vi "rozniczka.vi"(5 "dT":dbl format="%#_13g", 7 "u¿yj x0 (T)":bool=TRUE, 9 "Akcja (GET)":T1, 10 "x0":dbl format="%#_13g", 11 "Array in":dbl[](array[numeric])) -> (2 "ostatni":dbl, 3 "Array out":dbl[](array[numeric]))   [LabVIEW 2014]
uses:
  Kontrolki/FVGs/FVG akcje podstawowa.ctl
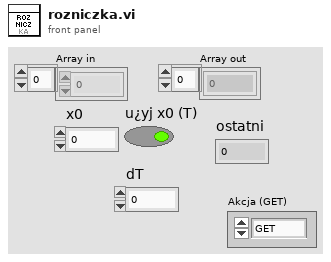
[diagram p1: front panel]
types:
  T1 = typedef "FVG akcje podstawowa.ctl" = enum16{"GET", "SET"}
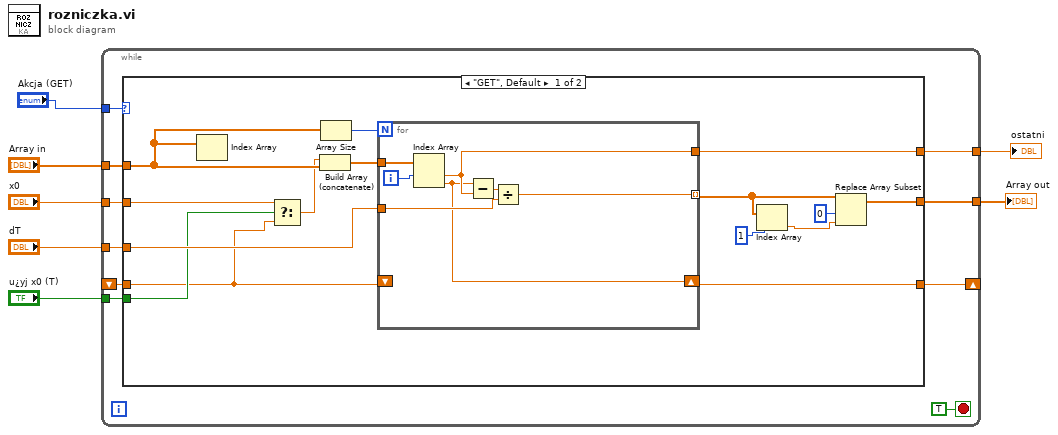
[diagram p0: block diagram]
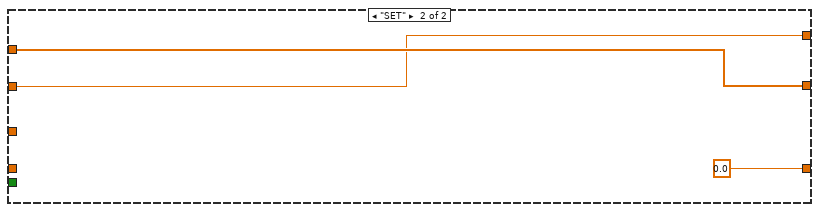
[diagram p2: hidden frame]
diagram:
  n1 = while {
    tunnel: "dT" -> [w17]
    tunnel: [w16] -> w6
    tunnel: "x0" -> [w14]
    tunnel: "u¿yj x0 (T)" -> [w13]
    tunnel: "Array in" -> [w15]
    tunnel: [w12] -> w2
    shift-right: [w10] -> _
    shift-left: _ -> [w9]
    tunnel: "Akcja (GET)" -> [w8]
    stop <- TRUE stop-if-true
    n2 = case shown="\"GET\", Default" w8 {
      tunnel: w17 -> [w30 _]
      tunnel: [w29 w40] -> w16
      tunnel: w15 -> [w28 w41]
      tunnel: w14 -> [w27 w40]
      tunnel: w13 -> [w25 _]
      tunnel: [w23 w41] -> w12
      tunnel: [w22 0.0] -> w10
      tunnel: w9 -> [w21 _]
      frame "GET", Default {
        n3 = Index Array(array=w28) -> ()  [unwired: 1 in, 1 out]
        n4 = Select(t=w27, s=w25, f=w21) -> (s? t:f=w26:dbl)
        n5 = Build Array (concatenate)(w26, w28) -> (w31:dbl[])
        n6 = Array Size(array=w28) -> (size(s)=w32:i32)
        n7 = for {
          N: w32 -> [_]
          tunnel: w31 -> [w39]
          tunnel: [w34] -> w24 mode=indexing
          tunnel: w30 -> [w36]
          tunnel: [w35] -> w29
          shift-right: [w33] -> w22
          shift-left: w21 -> [_]
          i -> [w38]
          n8 = Index Array(array=w39, index #1=w38) -> (element #1=w35:dbl, element #2=w33:dbl)  [unwired: 1 in]
          n9 = Subtract(x=w33, y=w35) -> (x-y=w37:dbl)
          n10 = Divide(x=w37, y=w36) -> (x/y=w34:dbl)
        }
        n11 = Index Array(array=w24, index=1) -> (element=w19:dbl)
        n12 = Replace Array Subset(array=w24, new element=w19, index=0) -> (w23:dbl[])
      }
      frame "SET" {
      }
    }
  }
  "Array out" <- w2
  "ostatni" <- w6
